vi "MakeFilename.vi"(9 "Numeric":i32, 10 "seconds since 1Jan1904":timestamp, 11 "created path":path) -> (3 "appended path":path)   [LabVIEW 2011]
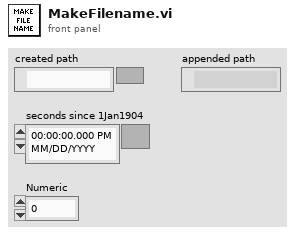
[diagram p1: front panel]
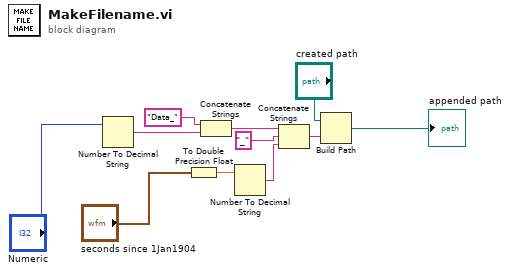
[diagram p0: block diagram]
diagram:
  n1 = Number To Decimal String(number="Numeric") -> (decimal integer string=w2:string)  [unwired: 1 in]
  n2 = To Double Precision Float(number="seconds since 1Jan1904") -> (double precision float=w6:dbl)
  n3 = Concatenate Strings("Data_" ("string"), w2) -> (w8:string)
  n4 = Number To Decimal String(number=w6) -> (decimal integer string=w7:string)  [unwired: 1 in]
  n5 = Concatenate Strings(w8, "_", w7) -> (w4:string)
  n6 = Build Path(base path="created path", name or relative path=w4) -> (appended path=→"appended path":path)
